vi "Run.vi"(8 "error in (no error)":errorcluster caption="entrée d'erreur (pas d'erreur)", 10 "Image":string[][](array[string]), 11 "Extract_Patches_2d.lvclass":refnum<class "Extract_Patches_2d.lvclass">) -> (0 "error out":errorcluster caption="sortie d'erreur", 2 "Data":T1, 3 "Extract_Patches_2d.lvclass":refnum<class "Extract_Patches_2d.lvclass">)   [LabVIEW 2020, in "Extract_Patches_2d.lvclass"]
doc: "Returns\n\n- patches : array of shape (n_patches, patch_height, patch_width) or (n_patches, patch_height, patch_width, n_channels)\nThe collection of patches extracted from the image, where n_patches is either max_patches or the total number of patches that can be extracted."
uses:
  Extract_Patches_2d.lvclass
  Extract_Patches_2d.lvclass/Extract_Patches_2d.ctl
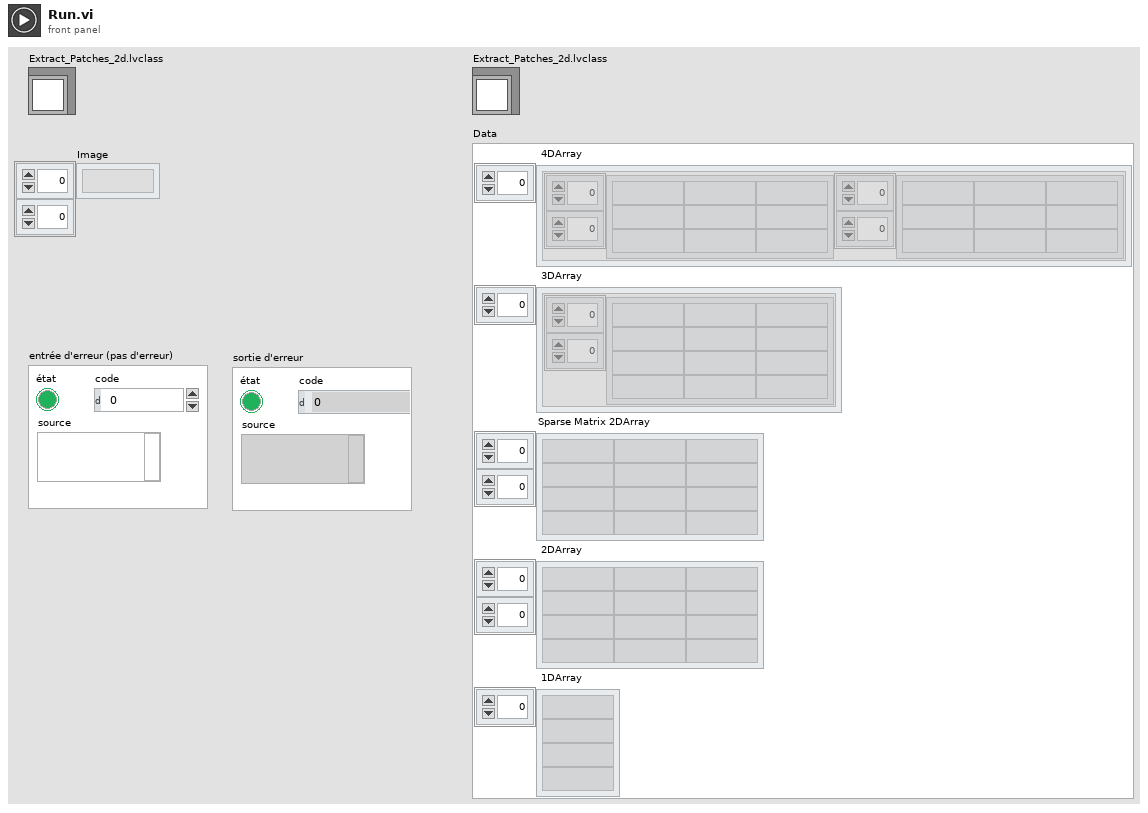
[diagram p1: front panel]
types:
  T1 = cluster{" 4DArray":cluster{"1":string[][], "2":string[][]}[], " 3DArray":cluster{"Tableau":string[][]}[], "Sparse Matrix 2DArray":string[][], " 2DArray":string[][], " 1DArray":string[]}
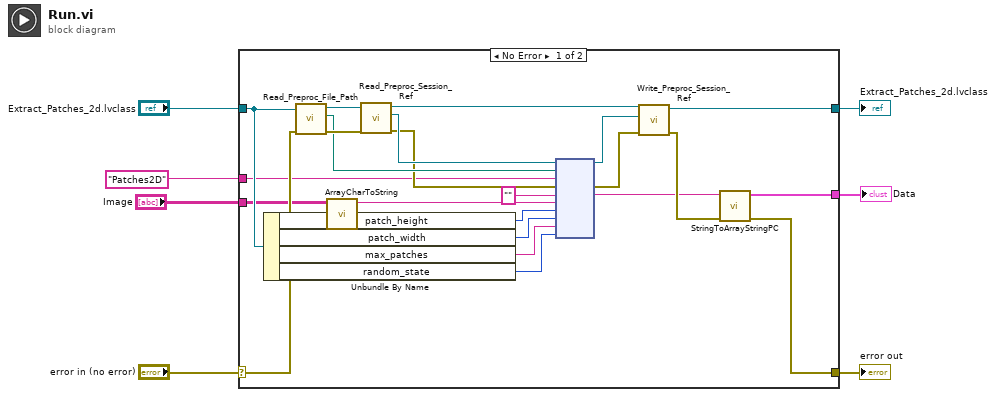
[diagram p0: block diagram]
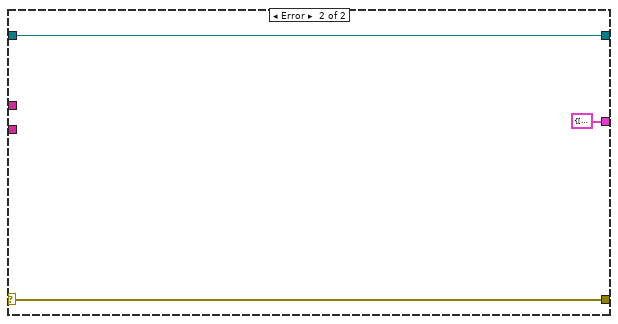
[diagram p2: hidden frame]
diagram:
  n1 = case shown="No Error" "error in (no error)" {
    selector: "error in (no error)" -> [w20 w33]
    tunnel: [w8 w33] -> w6
    tunnel: [w12 w32] -> w4
    tunnel: "Extract_Patches_2d.lvclass" -> [w21 w32]
    tunnel: "Patches2D" ("Fonction") -> [w19 _]
    tunnel: "Image" -> [w14 _]
    tunnel: [w9 T1 {" 4DArray"=[], " 3DArray"=[], "Sparse Matrix 2DArray"=[], " 2DArray"=[], " 1DArray"=[]} ("Data")] -> w1
    frame No Error {
      n2 = Unbundle By Name(w21) -> ("patch_height"=w18:i32, "patch_width"=w17:i32, "max_patches"=w16:string, "random_state"=w15:i32)
      n3 = call-dynamic "Read_Preproc_File_Path.vi"("error in (no error)"=w20, "Python in"=w21) -> ("error out"=w29:errorcluster, "File_Path"=w28:path, "Python out"=w30:refnum<class "Extract_Patches_2d.lvclass">)  [unwired: 7 in]
      n4 = call "ArrayCharToString.vi"("TAB"=w14) -> ("Instruction"=w13:string)  [unwired: 10 in]
      n5 = call-dynamic "Read_Preproc_Session_Ref.vi"("error in (no error)"=w29, "Python in"=w30) -> ("error out"=w26:errorcluster, "Session_ref"=w27:refnum<k35>, "Python out"=w25:refnum<class "Extract_Patches_2d.lvclass">)  [unwired: 7 in]
      n6 = node(w27, w28, w19, w26, "", w13, w18, w17, w16, w15) -> (w23:refnum<k35>, w24:errorcluster, w10:string)  [unwired: 5 in, 2 out]
      n7 = call-dynamic "Write_Preproc_Session_Ref.vi"("error in (no error)"=w24, "Session_ref"=w23, "Python in"=w25) -> ("error out"=w11:errorcluster, "Python out"=w12:refnum<class "Extract_Patches_2d.lvclass">)  [unwired: 7 in]
      n8 = call "StringToArrayStringPC.vi"("sortie d'erreur"=w11, "Return value"=w10) -> ("sortie d'erreur"=w8:errorcluster, "Data"=w9:T1)  [unwired: 8 in]
    }
    frame Error {
    }
  }
  "error out" <- w6
  "Extract_Patches_2d.lvclass" <- w4
  "Data" <- w1
